vi "Experiment_1.vi"() -> ()   [LabVIEW 2019]
uses:
  <vilib>/measure/maspectr.llb/FFT Spectrum (Mag-Phase) for N Chan.vi
  <vilib>/measure/maspectr.llb/FFT Spectrum (Mag-Phase) for 1 Chan.vi
  <vilib>/measure/NI_MABase.lvlib
  <vilib>/measure/NI_MAPro.lvlib
panel:
  out "Frequency spectrum of filtered random signal":cluster{"f0":dbl, "df":dbl, "magnitude":dbl[]}[](graph)
  out "Filtered random signal":dynamicdata(graph)
  out "Frequency spectrum of random signal":cluster{"f0":dbl, "df":dbl, "magnitude":dbl[]}(graph)
  out "Random Signal":waveform(dbl)(graph)
  in  "sampling info":cluster{"Fs":dbl, "#s":dbl}={"Fs"=1000.0, "#s"=1000.0} {"Fs" format="%.2p"}
  in  "amplitude":dbl=1.0 format="%.2p"
  in  "seed":i32=-1
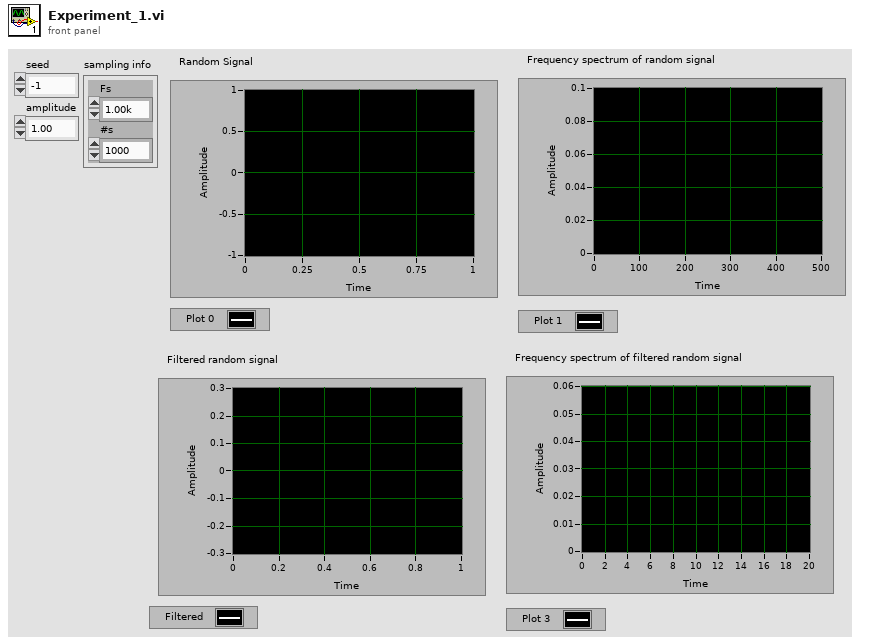
[diagram p1: front panel]
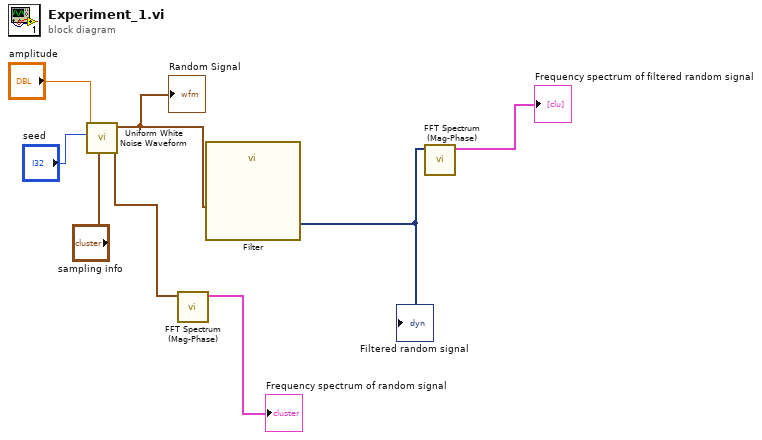
[diagram p0: block diagram]
diagram:
  n1 = call <vilib>:"Uniform White Noise Waveform.vi"("sampling info"="sampling info", "seed"="seed", "amplitude"="amplitude") -> ("signal out"=w4:waveform(dbl))  [unwired: 7 in, 1 out]
  "Random Signal" <- w4
  n2 = call-poly <vilib>:"FFT Spectrum (Mag-Phase).vi"("time signal"=w4) -> ("magnitude"=→"Frequency spectrum of random signal":cluster{"f0":dbl, "df":dbl, "magnitude":dbl[]})  [unwired: 6 in, 4 out]
  n3 = call "Filter"("Signal"=w4) -> ("Filtered Signal"=w2:dynamicdata)  [unwired: 9 in, 1 out]
  "Filtered random signal" <- w2
  n4 = call-poly <vilib>:"FFT Spectrum (Mag-Phase).vi"("time signals"=w2) -> ("magnitudes"=→"Frequency spectrum of filtered random signal":cluster{"f0":dbl, "df":dbl, "magnitude":dbl[]}[])  [unwired: 6 in, 4 out]
